vi "autonomousinfo.vi"() -> ()   [LabVIEW 2020]
doc: "These global variables report autonomous sequencing and path following data."
panel:
  out "Auto_Force_To_High_Gear":bool
  out "Auto_Preload_Balls":i32
  out "Auto_Intake_On":bool
  out "Robot_is_Pathing":bool
  out "Auto_Rumble_Driver_Joystick":bool
  out "Auto_Spin_Shooter":bool
  out "Auto_Path_Suffix":string
  out "Auto_Error":errorcluster
  out "Distance_From_Start (in)":dbl
  out "Distance_From_End (in)":dbl
  out "Auto_Manipulator_Step":i32
  out "Auto_Drive_Step":i32
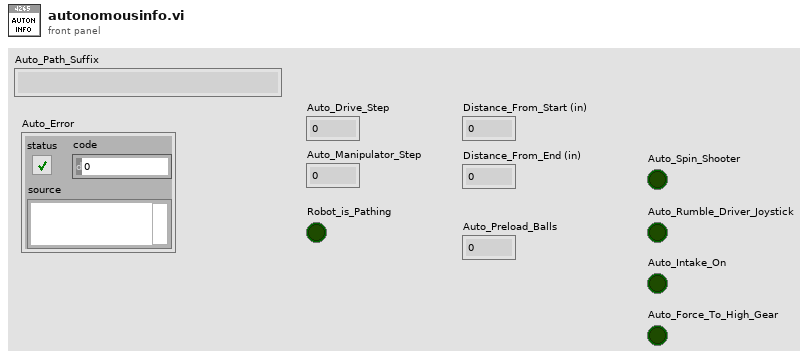
[diagram p1: front panel]
diagram:
